vi "Reset.vi"(7 "Slave Address":i32=-1 min=-1 max=30 step=1, 8 "error":errorcluster, 9 "Settle (0 mS)":u32, 10 "Reset (T)":bool=TRUE, 11 "VISA":refnum<visa-resource-name>) -> (0 "error out":errorcluster, 3 "VISA out":refnum<visa-resource-name>)   [LabVIEW 2025, in "TDK-Lambda GEN LAN Series.lvlib"]
doc: "Resets the GEN power supply to a known and safe state, if the Reset control is set TRUE (default). This VI will wait for \"Settle\" milliseconds after Reset to allow the output to turn off.\n\nThe reset state includes:\n- Output off\n- Voltage and current program limits to zero\n- Safe-start is enabled\n- Over-voltage protection setting to maximum\n- Under-voltage limit to zero\n- Fold-back protection off"
uses:
  <userlib>/TDK-Lambda GEN LAN Series/TDK-Lambda GEN LAN Series.lvlib
panel:
  # "TDK-Lambda Genesys \n LAN\n  DC Power Supplies"
  # "Reset Power Supply"
  # "(c) 2019 TDK-Lambda.  ALL RIGHTS RESERVED."
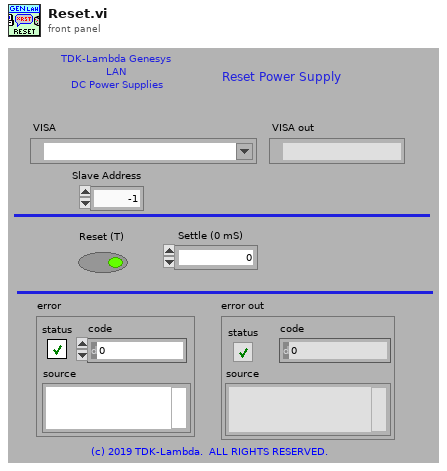
[diagram p1: front panel]
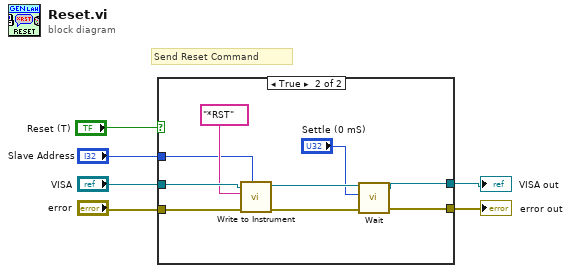
[diagram p0: block diagram]
diagram:
  # "Send Reset Command"
  n1 = case shown="True" "Reset (T)" {
    tunnel: "VISA" -> [w8 w17]
    tunnel: [w8 w13] -> w5
    tunnel: "error" -> [w7 w16]
    tunnel: [w7 w12] -> w3
    tunnel: "Slave Address" -> [_ w9]
    frame False {
    }
    frame True {
      n2 = call <userlib>:"Write to Instrument.vi"("Slave Address"=w9, "error"=w16, "Command"="*RST", "VISA"=w17) -> ("error out"=w11:errorcluster, "VISA out"=w14:refnum<visa-resource-name>)  [unwired: 6 in]
      n3 = call <userlib>:"Wait.vi"("error"=w11, "Delay (20 mS)"="Settle (0 mS)", "VISA"=w14) -> ("error out"=w12:errorcluster, "VISA out"=w13:refnum<visa-resource-name>)  [unwired: 7 in]
    }
  }
  "VISA out" <- w5
  "error out" <- w3
